vi "PR_Write_tracker_stream_to_TDMS.vi"(8 "error in (no error)":errorcluster, 10 "Data in":T2, 11 "TDMS ref. in":refnum<k34>) -> (0 "error out":errorcluster)   [LabVIEW 2018, in "Tracker.lvlib"]
uses:
  Tracker.lvlib
  Controls/CTL_Animal_Coordinates_and_Speed.ctl
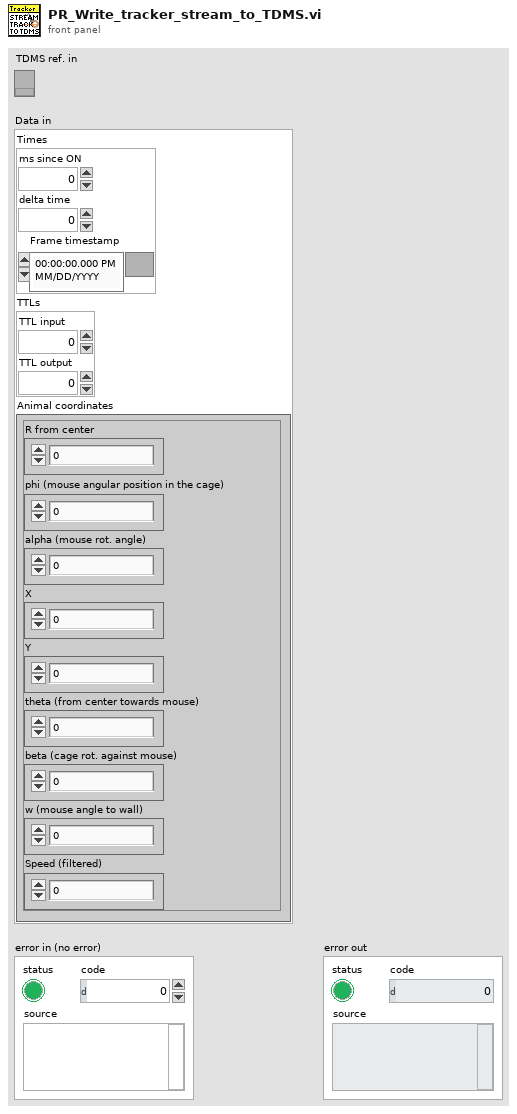
[diagram p1: front panel]
types:
  T1 = typedef "Tracker.lvlib/CTL_Animal_Coordinates_and_Speed.ctl" = cluster{"R from center":dbl, "phi (mouse angular position in the cage)":dbl, "alpha (mouse rot. angle)":sgl, "X":dbl, "Y":dbl, "theta (from center towards mouse)":dbl, "beta (cage rot. against mouse)":sgl, "w (mouse angle to wall)":dbl, "Speed (filtered)":dbl}
  T2 = cluster{"Times":cluster{"ms since ON":u32, "delta time":u32, "Frame timestamp":timestamp}, "TTLs":cluster{"TTL input":i16, "TTL output":i16}, "Animal coordinates":T1}
  T3 = cluster{"ms since ON":u32, "delta time":u32, "Frame timestamp":timestamp}
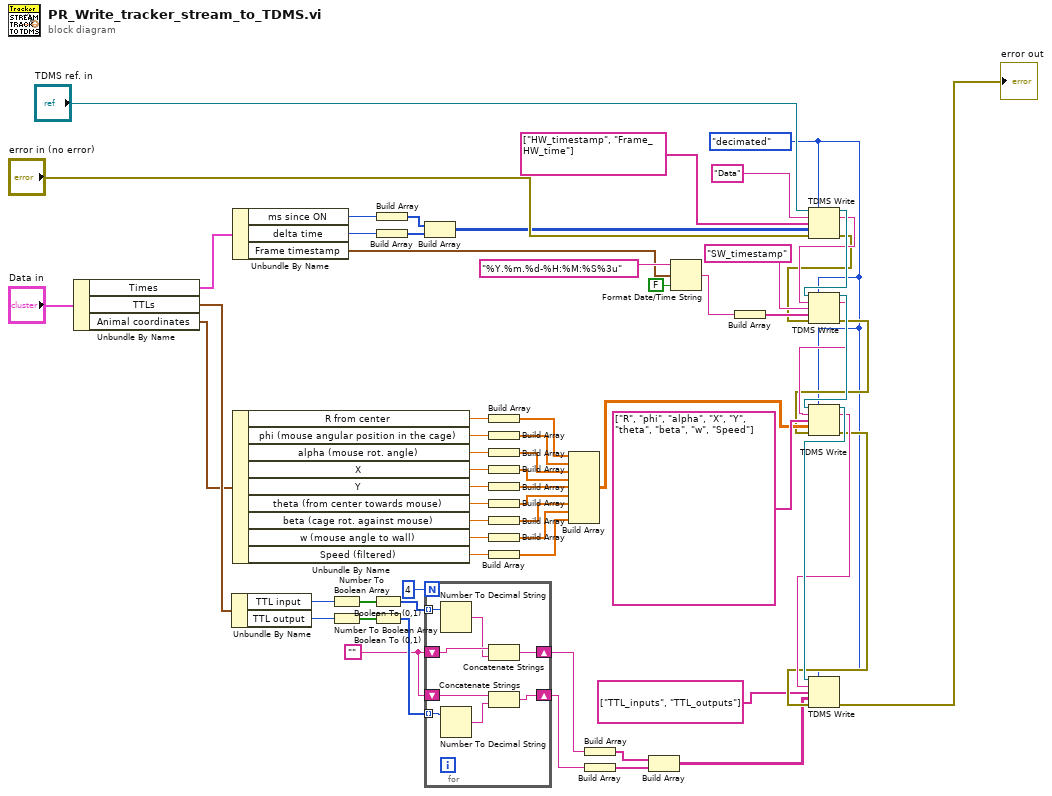
[diagram p0: block diagram]
diagram:
  w6 = ""
  w9 = enum16{"decimated", "interleaved"}."decimated" ("data layout (0:decimated)")
  n1 = Unbundle By Name("Data in") -> ("Times"=w63:T3, "TTLs"=w62:cluster{"TTL input":i16, "TTL output":i16}, "Animal coordinates"=w61:T1)
  n2 = Unbundle By Name(w62) -> ("TTL input"=w14:i16, "TTL output"=w13:i16)
  n3 = Unbundle By Name(w63) -> ("ms since ON"=w56:u32, "delta time"=w55:u32, "Frame timestamp"=w50:timestamp)
  n4 = Unbundle By Name(w61) -> ("R from center"=w42:dbl, "phi (mouse angular position in the cage)"=w41:dbl, "alpha (mouse rot. angle)"=w40:sgl, "X"=w39:dbl, "Y"=w38:dbl, "theta (from center towards mouse)"=w37:dbl, "beta (cage rot. against mouse)"=w36:sgl, "w (mouse angle to wall)"=w35:dbl, "Speed (filtered)"=w34:dbl)
  n5 = Number To Boolean Array(number=w14) -> (Boolean array=w15:bool[])
  n6 = Number To Boolean Array(number=w13) -> (Boolean array=w11:bool[])
  n7 = Boolean To (0,1)(Boolean=w15) -> (0, 1=w7:i16[])
  n8 = Boolean To (0,1)(Boolean=w11) -> (0, 1=w10:i16[])
  n9 = Build Array(w56) -> (w53:u32[])
  n10 = Build Array(w55) -> (w52:u32[])
  n11 = Build Array(w53, w52) -> (w54:u32[][])
  n12 = for {
    N: 4 -> [_]
    tunnel: w10 -> [w72] mode=indexing
    tunnel: w7 -> [w71] mode=indexing
    shift-right: [w70] -> w5
    shift-left: w6 -> [w69]
    shift-right: [w66] -> w4
    shift-left: w6 -> [w65]
    n13 = Number To Decimal String(number=w71) -> (decimal integer string=w68:string)  [unwired: 1 in]
    n14 = Number To Decimal String(number=w72) -> (decimal integer string=w67:string)  [unwired: 1 in]
    n15 = Concatenate Strings(w69, w68) -> (w70:string)
    n16 = Concatenate Strings(w65, w67) -> (w66:string)
  }
  n17 = Build Array(w42) -> (w33:dbl[])
  n18 = Build Array(w41) -> (w32:dbl[])
  n19 = Build Array(w40) -> (w31:sgl[])
  n20 = Build Array(w39) -> (w30:dbl[])
  n21 = Build Array(w38) -> (w29:dbl[])
  n22 = Build Array(w37) -> (w28:dbl[])
  n23 = Build Array(w36) -> (w27:sgl[])
  n24 = Build Array(w35) -> (w26:dbl[])
  n25 = Build Array(w34) -> (w25:dbl[])
  n26 = Build Array(w33, w32, w31, w30, w29, w28, w27, w26, w25) -> (w21:dbl[][])
  n27 = Build Array(w5) -> (w3:string[])
  n28 = Build Array(w4) -> (w2:string[])
  n29 = Build Array(w3, w2) -> (w8:string[][])
  n30 = Format Date/Time String(time format string (%c)="%Y.%m.%d-%H:%M:%S%3u", seconds (now)=w50, UTC format=FALSE) -> (date/time string=w46:string)
  n31 = Build Array(w46) -> (w45:string[])
  n32 = TDMS Write(0:"TDMS ref. in", 1:w9, 5:"Data" ("group name in (Untitled)"), 7:string[] ["HW_timestamp", "Frame_HW_time"] ("channel name(s) in (Untitled)"), 9:w54, 11:"error in (no error)") -> (4:w48:refnum<k34>, 6:w47:string, 15:w43:errorcluster)  [unwired: 1 out]
  n33 = TDMS Write(0:w48, 1:w9, 5:w47, 7:"SW_timestamp" ("channel name(s) in (Untitled)"), 9:w45, 11:w43) -> (4:w24:refnum<k34>, 6:w23:string, 15:w20:errorcluster)  [unwired: 1 out]
  n34 = TDMS Write(0:w24, 1:w9, 5:w23, 7:string[] ["R", "phi", "alpha", "X", "Y", "theta", "beta", "w", "Speed"] ("appended array"), 9:w21, 11:w20) -> (4:w19:refnum<k34>, 6:w18:string, 15:w17:errorcluster)  [unwired: 1 out]
  n35 = TDMS Write(0:w19, 1:w9, 5:w18, 7:string[] ["TTL_inputs", "TTL_outputs"] ("channel name(s) in (Untitled)"), 9:w8, 11:w17) -> (15:→"error out":errorcluster)  [unwired: 3 out]
